vi "雷达.vi"(5 "错误输入（无错误）":errorcluster, 6 "VISA资源名称":refnum<visa-resource-name>) -> (0 "位置信息":cluster{dbl, dbl}, 1 "指示灯":cluster{bool, bool, bool}, 2 "Polar Plot":picture caption="极坐标图", 3 "VISA资源名称输出":refnum<visa-resource-name>, 4 "错误输出":errorcluster)   [LabVIEW 2018]
panel:
  out "字符串":string
  out "字符串 2":string
  out "连接的字符串 2":string
  out "连接的字符串":string
  out "响应":string
  in  "等待时间（毫秒）":u32
  in  "命令":string="*IDN?"
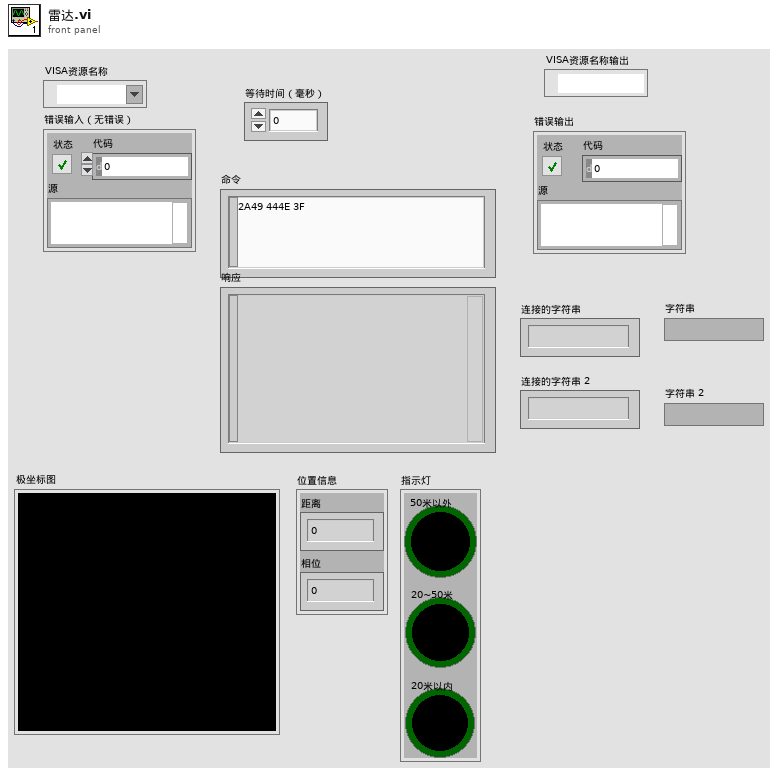
[diagram p1: front panel]
types:
  T1 = cluster{"maximum":dbl, "minimum":dbl, "clip to min":bool, "log?(F)":bool, "grid color":u32, "plot color":u32, "fmt and prec":cluster{"format":enum8{"Decimal", "Scientific", "Engineering", "Binary", "Octal", "Hex"}, "precision":u8}, "visible section":u16}
  T2 = typedef "LVBoundsTypeDef.ctl" = cluster{"Width":u32, "Height":u32}
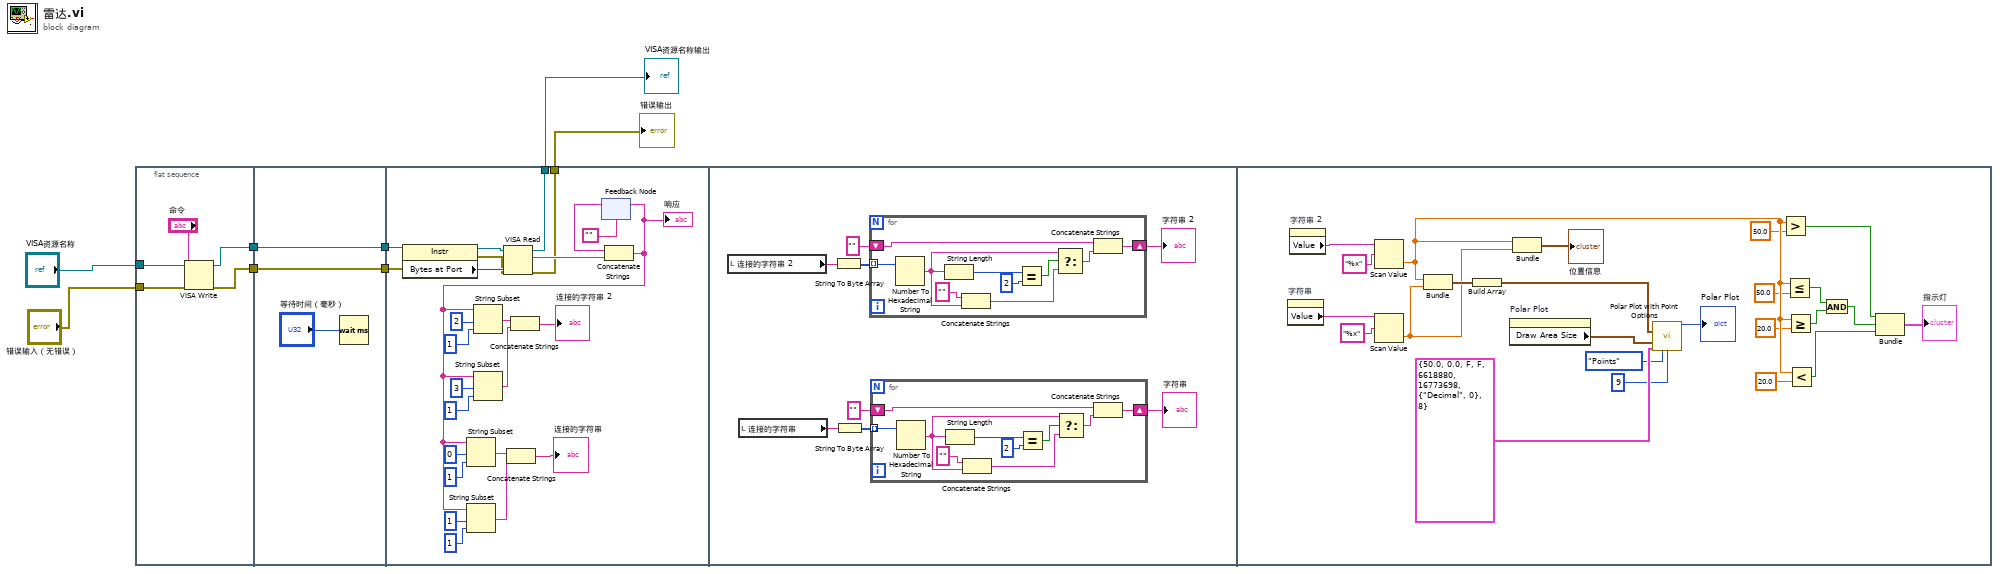
[diagram p0: block diagram]
diagram:
  n1 = flat-sequence {
    tunnel: [w13] -> w8
    tunnel: [w12] -> w7
    tunnel: "VISA资源名称" -> [w10]
    tunnel: "错误输入（无错误）" -> [w9]
    tunnel: w8 -> [w16]
    tunnel: [w16] -> w6
    tunnel: w7 -> [w15]
    tunnel: [w15] -> w5
    tunnel: w6 -> [w37]
    tunnel: w5 -> [w36]
    tunnel: [w18] -> w4
    tunnel: [w17] -> w3
    frame #0 {
      n2 = VISA Write(VISA resource name=w10, write buffer="命令", error in (no error)=w9) -> (VISA resource name out=w13:refnum<visa-resource-name>, error out=w12:errorcluster)  [unwired: 1 out]
    }
    frame #1 {
      n3 = Wait (ms)(milliseconds to wait="等待时间（毫秒）") -> ()  [unwired: 1 out]
    }
    frame #2 {
      n4 = property class="Instr"(reference=w37, error in=w36) -> (reference out=w39:refnum<visa-resource-name>, error out=w40:errorcluster, "Bytes at Port"=w41:u32)
      n5 = VISA Read(VISA resource name=w39, byte count=w41, error in (no error)=w40) -> (VISA resource name out=w18:refnum<visa-resource-name>, read buffer=w20:string, error out=w17:errorcluster)  [unwired: 1 out]
      n6 = feedback #1("") -> (w38:string)
      n7 = Concatenate Strings(w38, w20) -> (w19:string)
      "响应" <- w19
      n8 = String Subset(string=w19, offset (0)=0 ("偏移量(0)"), length (rest)=1 ("长度（剩余）")) -> (substring=w33:string)
      n9 = String Subset(string=w19, offset (0)=1 ("偏移量(0)"), length (rest)=1 ("长度（剩余）")) -> (substring=w32:string)
      n10 = String Subset(string=w19, offset (0)=2 ("偏移量(0)"), length (rest)=1 ("长度（剩余）")) -> (substring=w31:string)
      n11 = String Subset(string=w19, offset (0)=3 ("偏移量(0)"), length (rest)=1 ("长度（剩余）")) -> (substring=w30:string)
      n12 = Concatenate Strings(w33, w32) -> (→"连接的字符串":string)
      n13 = Concatenate Strings(w31, w30) -> (→"连接的字符串 2":string)
      n14 = feedback-in #1(w19) -> ()
    }
    frame #3 {
      n15 = local read "连接的字符串 2"() -> (w47:string)
      n16 = local read "连接的字符串"() -> (w44:string)
      n17 = String To Byte Array(string=w47) -> (unsigned byte array=w49:u8[])
      n18 = String To Byte Array(string=w44) -> (unsigned byte array=w45:u8[])
      n19 = for {
        shift-right: [w60] -> w48
        shift-left: "" -> [w62]
        tunnel: w49 -> [w69] mode=indexing
        n20 = Number To Hexadecimal String(2:w69) -> (0:w63:string)  [unwired: 1 in]
        n21 = String Length(string=w63) -> (length=w68:i32)
        n22 = Concatenate Strings("" ("字符串"), w63) -> (w64:string)
        n23 = Equal?(x=w68, y=2) -> (x = y?=w66:bool)
        n24 = Select(t=w63, s=w66, f=w64) -> (s? t:f=w61:string)
        n25 = Concatenate Strings(w62, w61) -> (w60:string)
      }
      "字符串 2" <- w48
      n26 = for {
        shift-right: [w50] -> w43
        shift-left: "" -> [w52]
        tunnel: w45 -> [w59] mode=indexing
        n27 = Number To Hexadecimal String(2:w59) -> (0:w53:string)  [unwired: 1 in]
        n28 = String Length(string=w53) -> (length=w58:i32)
        n29 = Concatenate Strings("" ("字符串"), w53) -> (w54:string)
        n30 = Equal?(x=w58, y=2) -> (x = y?=w56:bool)
        n31 = Select(t=w53, s=w56, f=w54) -> (s? t:f=w51:string)
        n32 = Concatenate Strings(w52, w51) -> (w50:string)
      }
      "字符串" <- w43
    }
    frame #4 {
      n33 = property on="字符串" class="Str"() -> ("Value"=w88:string)  [unwired: 2 in, 2 out]
      n34 = property on="字符串 2" class="Str"() -> ("Value"=w89:string)  [unwired: 2 in, 2 out]
      n35 = Scan Value(string=w89, format string="%x" ("格式字符串")) -> (value=w85:dbl)  [unwired: 1 in, 1 out]
      n36 = Scan Value(string=w88, format string="%x" ("格式字符串")) -> (value=w84:dbl)  [unwired: 1 in, 1 out]
      n37 = Bundle(w85, w84) -> (w92:cluster{dbl, dbl})  [unwired: 1 in]
      n38 = Build Array(w92) -> (w93:cluster{dbl, dbl}[])
      n39 = property on="Polar Plot" class="Pict"() -> ("Draw Area Size"=w91:T2)  [unwired: 2 in, 2 out]
      n40 = Bundle(w85, w84) -> (→"位置信息":cluster{dbl, dbl})  [unwired: 1 in]
      n41 = call <vilib>:"Polar Plot with Point Options.vi"("data array [mag, phase (deg)]"=w93, "dimensions (w,h)"=w91, "polar attributes"=T1 {"maximum"=50.0, "minimum"=0.0, "clip to min"=FALSE, "log?(F)"=FALSE, "grid color"=6618880, "plot color"=16773698, "fmt and prec"={"format"=enum."Decimal", "precision"=0}, "visible section"=8}, "Lines/Points"=enum16{"Lines", "Points"}."Points", "Size"=u16 9) -> ("new picture"=→"Polar Plot":picture)  [unwired: 10 in]
      n42 = Greater?(x=w85, y=50.0) -> (0:w82:bool)
      n43 = Less Or Equal?(x=w85, y=50.0) -> (x <= y?=w86:bool)
      n44 = Greater Or Equal?(x=w85, y=20.0) -> (x >= y?=w87:bool)
      n45 = Less?(x=w85, y=20.0) -> (x < y?=w80:bool)
      n46 = And(x=w86, y=w87) -> (x .and. y?=w81:bool)
      n47 = Bundle(w82, w81, w80) -> (→"指示灯":cluster{bool, bool, bool})  [unwired: 1 in]
    }
  }
  "VISA资源名称输出" <- w4
  "错误输出" <- w3
